vi "pairClient.vi"() -> ()   [LabVIEW 2014]
uses:
  <vilib>/addons/zeromq/socket_type.ctl
  <vilib>/addons/zeromq/zmq_context.lvclass
  <vilib>/addons/zeromq/zeromq.lvlib
  <vilib>/addons/zeromq/zmq_socket.lvclass
panel:
  out "concatenated string":string
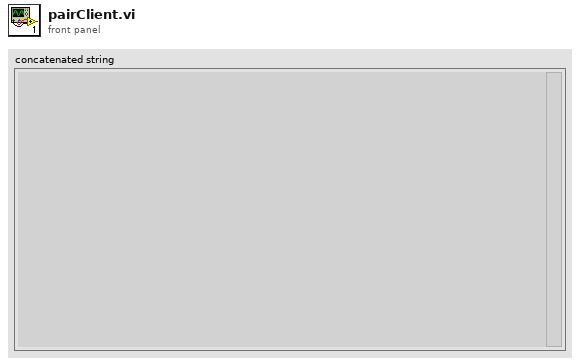
[diagram p1: front panel]
types:
  T1 = typedef "zeromq.lvlib/socket_type.ctl" = enum8{"ZMQ_PAIR", "ZMQ_PUB", "ZMQ_SUB", "ZMQ_REQ", "ZMQ_REP", "ZMQ_DEALER", "ZMQ_ROUTER", "ZMQ_PULL", "ZMQ_PUSH", "ZMQ_XPUB", "ZMQ_XSUB"}
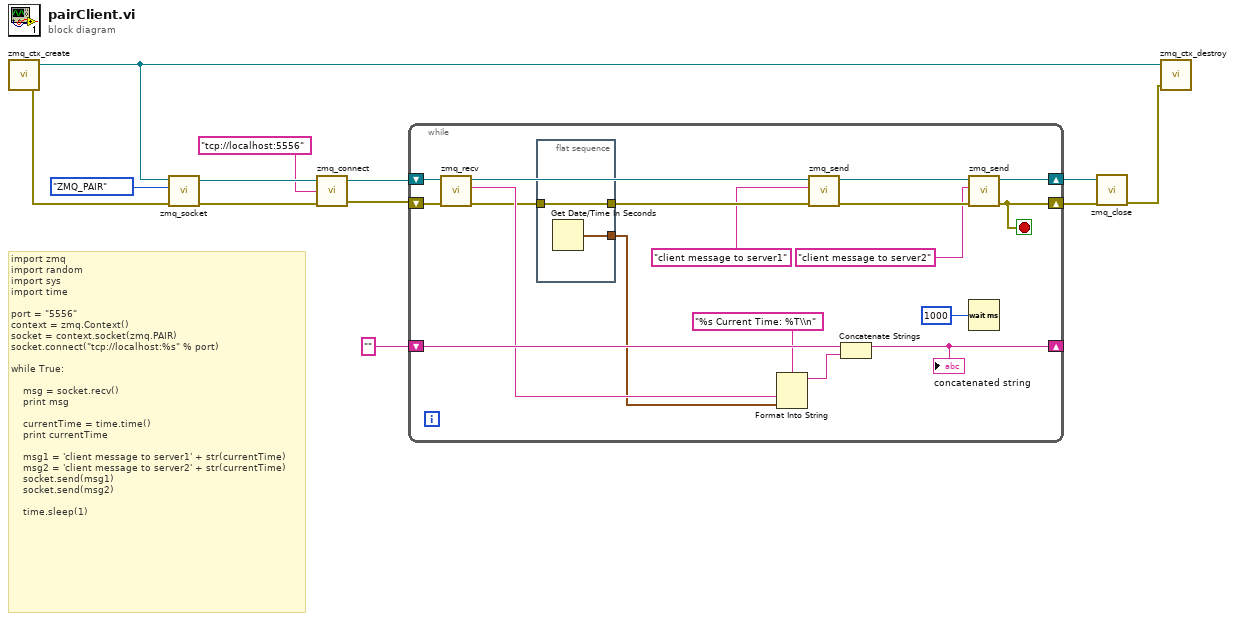
[diagram p0: block diagram]
diagram:
  # "import zmq\nimport random\nimport sys\nimport time\n\nport = \"5556\"\ncontext = zmq.Context()\nsocket = context.socket(zmq.PAIR)\nsocket.connect(\"tcp://localhost:%s\" % port)\n\nwhile True:\n\n    msg = socket.recv()\n    print msg\n\n    currentTime = time.time()\n    print currentTime\n\n    msg1 = 'client message to server1' + str(currentTime)\n    msg2 = 'client message to server2' + str(currentTime)\n    socket.send(msg1)\n    socket.send(msg2)\n\n    time.sleep(1)"
  n1 = call <vilib>:"zmq_ctx_create.vi"() -> ("error out"=w11:errorcluster, "context out"=w10:refnum<class "zmq_context.lvclass">)  [unwired: 4 in]
  n2 = call <vilib>:"zmq_socket.vi"("error in"=w11, "socket type"=socket_type."ZMQ_PAIR", "context in"=w10) -> ("error out"=w8:errorcluster, "socket out"=w9:refnum<class "zmq_socket.lvclass">)  [unwired: 2 in, 1 out]
  n3 = call <vilib>:"zmq_connect.vi"("error in"=w8, "endpoint"="tcp://localhost:5556", "socket in"=w9) -> ("error out"=w5:errorcluster, "socket out"=w6:refnum<class "zmq_socket.lvclass">)  [unwired: 1 in]
  n4 = while {
    shift-right: [w17] -> w4
    shift-left: w6 -> [w30]
    shift-right: [w13] -> w3
    shift-left: w5 -> [w29]
    shift-right: [w25] -> _
    shift-left: "" -> [w27]
    stop <- w13 stop-if-true
    n5 = call <vilib>:"zmq_recv.vi"("error in"=w29, "socket in"=w30) -> ("error out"=w20:errorcluster, "data"=w23:string, "socket out"=w28:refnum<class "zmq_socket.lvclass">)  [unwired: 3 in, 2 out]
    n6 = flat-sequence {
      tunnel: [w32] -> w22
      tunnel: [w31] -> w21
      tunnel: w20 -> [w31]
      frame #0 {
        n7 = Get Date/Time In Seconds() -> (seconds since 1Jan1904=w32:timestamp)
      }
    }
    n8 = Format Into String(format string="%s Current Time: %T\\n", w23, w22) -> (resulting string=w24:string)  [unwired: 2 in, 1 out]
    n9 = call <vilib>:"zmq_send.vi"("error in"=w21, "data"="client message to server1", "socket in"=w28) -> ("error out"=w19:errorcluster, "socket out"=w18:refnum<class "zmq_socket.lvclass">)  [unwired: 4 in]
    n10 = Concatenate Strings(w27, w24) -> (w25:string)
    "concatenated string" <- w25
    n11 = call <vilib>:"zmq_send.vi"("error in"=w19, "data"="client message to server2", "socket in"=w18) -> ("error out"=w13:errorcluster, "socket out"=w17:refnum<class "zmq_socket.lvclass">)  [unwired: 4 in]
    n12 = Wait (ms)(milliseconds to wait=u32 1000) -> ()  [unwired: 1 out]
  }
  n13 = call <vilib>:"zmq_close.vi"("error in"=w3, "socket"=w4) -> ("error out"=w2:errorcluster)  [unwired: 3 in]
  n14 = call <vilib>:"zmq_ctx_destroy.vi"("error in"=w2, "context in"=w10) -> ()  [unwired: 3 in, 1 out]
